vi "Write Sink Settings.vi"(0 "Event Source in":refnum<class "Event Source.lvclass">, 1 "Sink Name":string, 3 "Sink Settings":T1, 5 "error in (no error)":errorcluster) -> (14 "Event Source out":refnum<class "Event Source.lvclass">, 19 "error out":errorcluster)   [LabVIEW 2016, in "Event Source.lvlib" / "Event Source.lvclass"]
doc: "Allows to set the Sink behaviour by setting the following flags\n\n\"Exclude From Broadcast\"\nmessage originating form another sink will not be broadcasted to the sink being cosidered\n\"Paused\"\nThe sink will not send events and will not receive them anymore\n\"Receive only\"\nThe sing will receive events but not sany any"
uses:
  Event Source.lvclass
  Sink Settings.ctl
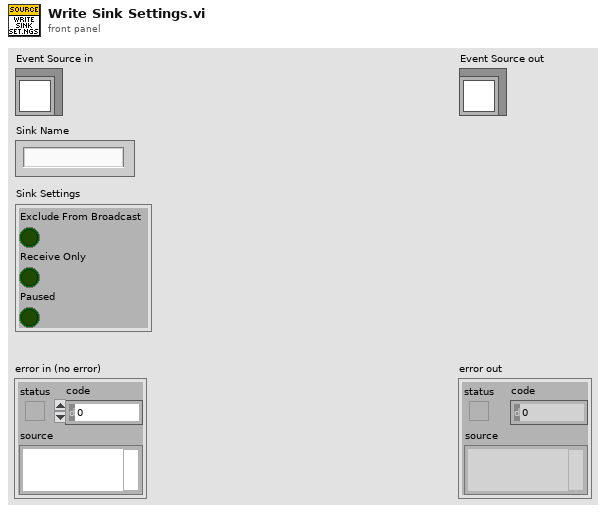
[diagram p1: front panel]
types:
  T1 = typedef "Event Source.lvlib/Event Source.lvclass/Sink Settings.ctl" = cluster{"Exclude From Broadcast":bool, "Receive Only":bool, "Paused":bool}
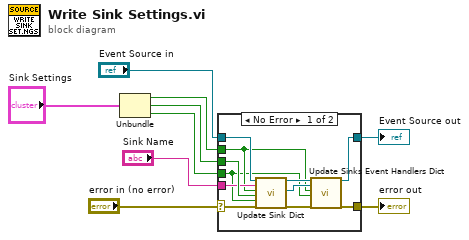
[diagram p0: block diagram]
diagram:
  n1 = Unbundle("Sink Settings") -> ("Exclude From Broadcast"=w3:bool, "Receive Only"=w1:bool, "Paused"=w2:bool)
  n2 = case shown="No Error" "error in (no error)" {
    selector: "error in (no error)" -> [w20 w22]
    tunnel: [w15 w22] -> w8
    tunnel: [w13 w21] -> w6
    tunnel: "Event Source in" -> [w19 w21]
    tunnel: "Sink Name" -> [w17 _]
    tunnel: w3 -> [w11 _]
    tunnel: w1 -> [w18 _]
    tunnel: w2 -> [w10 _]
    frame No Error {
      n3 = call "Update Sink Dict.vi"("Event Source in"=w19, "Sink Name"=w17, "Exclude From Broadcast (F)"=w11, "Receive Only (F)"=w18, "Paused (F)"=w10, "error in (no error)"=w20) -> ("Event Source out"=w14:refnum<class "Event Source.lvclass">, "Sink Enququer"=w12:refnum<class "Message Enqueuer.lvclass">, "error out"=w16:errorcluster)  [unwired: 11 in]
      n4 = call "Update Sinks Event Handlers Dict.vi"("Event Source in"=w14, "Sink Enququer"=w12, "Exclude From Broadcast (F)"=w11, "Paused (F)"=w10, "error in (no error)"=w16) -> ("Event Source out"=w13:refnum<class "Event Source.lvclass">, "error out"=w15:errorcluster)  [unwired: 13 in]
    }
    frame Error {
    }
  }
  "error out" <- w8
  "Event Source out" <- w6
